vi "FTW-CodeGen-Bounds.vi"(0 "State In":T1 {"Actor Interface"."Bounds"."Left" format="%dpx"; "Actor Interface"."Bounds"."Top" format="%dpx"; "Actor Interface"."Bounds"."Right" format="%dpx"; "Actor Interface"."Bounds"."Bottom" format="%dpx"}, 5 "XRef":refnum<vi>) -> (4 "Bounds":cluster{"Width":i32, "Height":i32})   [LabVIEW 2014, in "FTW-Actor-Spawn.xnode"]
uses:
  FTW-Actor-Spawn.xnode
  FTW-CodeGen-State.ctl
panel:
  # "Inputs"
  # "Outputs"
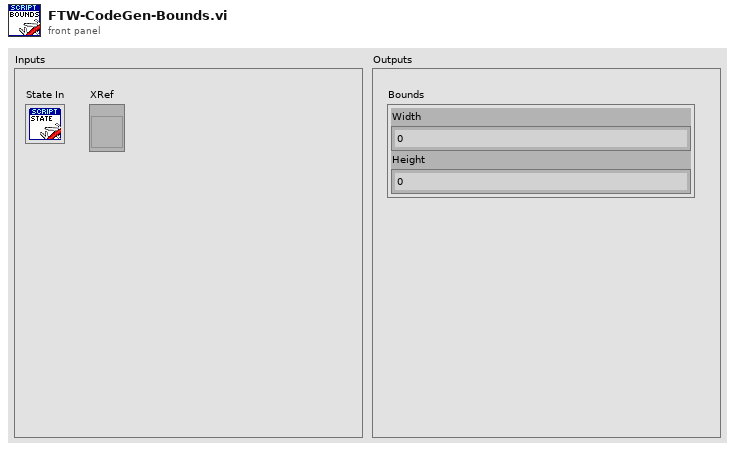
[diagram p1: front panel]
types:
  T1 = typedef "FTW-Actor-Spawn.xnode/FTW-CodeGen-State.ctl" = cluster{"Path Wired?":bool, "Actor Interface":cluster{"Name":string, "Type":variant, "Bounds":cluster{"Left":i32, "Top":i32, "Right":i32, "Bottom":i32}, "Input":bool, "Recommended":bool, "Required":bool, "Dynamic Dispatch":bool, "On Interface":bool, "\"The\" Config Terminal":bool}[], "Config Terminal Index":i32}
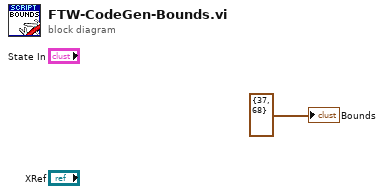
[diagram p0: block diagram]
diagram:
  "Bounds" <- cluster{"Width":i32, "Height":i32} {"Width"=37, "Height"=68} ("Bounds")
